vi "As PropertyObjectFile.vi"(8 "error in (no error)":errorcluster, 11 "SequenceFile in":refnum<class "SequenceFile.lvclass">) -> (0 "error out":errorcluster, 2 "PropertyObjectFile":refnum<k7>, 3 "SequenceFile out":refnum<class "SequenceFile.lvclass">)   [LabVIEW 2020, in "TSnax.lvlib" / "SequenceFile.lvclass"]
uses:
  SequenceFile.lvclass
  SequenceFile.lvclass/SequenceFile.ctl
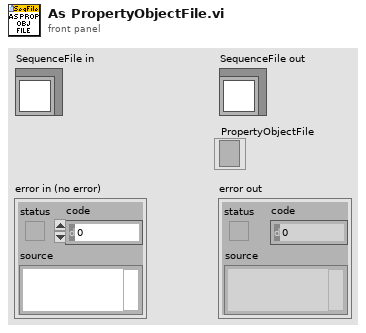
[diagram p1: front panel]
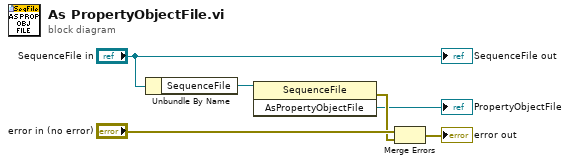
[diagram p0: block diagram]
diagram:
  n1 = Unbundle By Name("SequenceFile in") -> ("SequenceFile"=w4:refnum<k7>)
  n2 = invoke class="SequenceFile" method="AsPropertyObjectFile"(reference=w4) -> (error out=w2:errorcluster, "AsPropertyObjectFile"=→"PropertyObjectFile":refnum<k7>)  [unwired: 2 in, 1 out]
  n3 = Merge Errors("error in (no error)", w2) -> (→"error out":errorcluster)
  "SequenceFile out" <- "SequenceFile in"
